vi "Write Test VI Name.vi"(8 "error in":errorcluster, 10 "Test VI Name":string, 11 "Naming Data in":refnum<class "Naming Data.lvclass">) -> (0 "error out":errorcluster, 3 "Naming Data out":refnum<class "Naming Data.lvclass">)   [LabVIEW 2020, in "Approval Tests.lvlib" / "Naming Data.lvclass"]
uses:
  Naming Data.lvclass
  Naming Data.lvclass/Naming Data.ctl
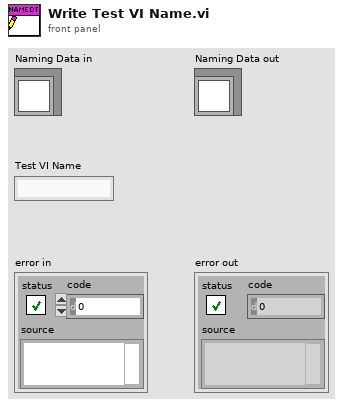
[diagram p1: front panel]
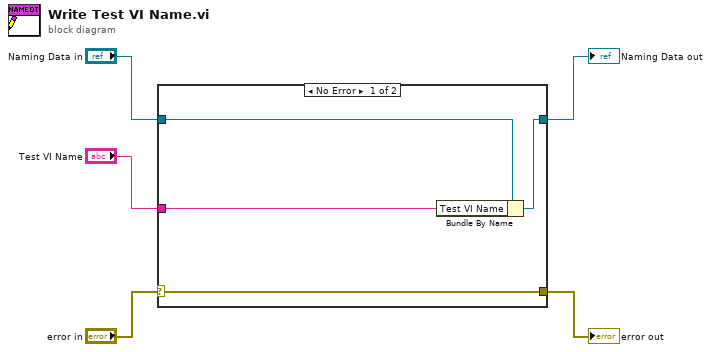
[diagram p0: block diagram]
diagram:
  n1 = case shown="No Error" "error in" {
    selector: "error in" -> [w9 w11]
    tunnel: [w9 w11] -> w4
    tunnel: [w7 w10] -> w2
    tunnel: "Naming Data in" -> [w8 w10]
    tunnel: "Test VI Name" -> [w6 _]
    frame No Error {
      n2 = Bundle By Name(cluster=w8, "Test VI Name"=w6) -> (w7:refnum<class "Naming Data.lvclass">)
    }
    frame Error {
    }
  }
  "error out" <- w4
  "Naming Data out" <- w2
